vi "FtoC_SubVI.vi"(1 "Temperatura a Convertir":dbl) -> (0 "Temperatura Convertida":dbl)   [LabVIEW 2013]
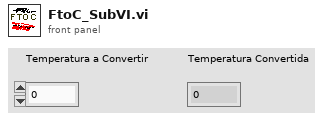
[diagram p1: front panel]
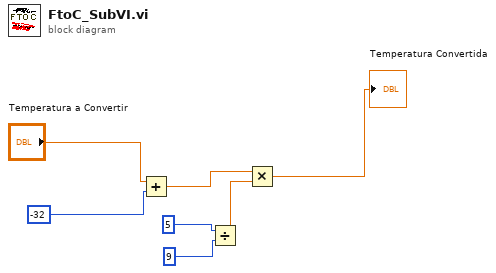
[diagram p0: block diagram]
diagram:
  n1 = Add(x="Temperatura a Convertir", y=-32) -> (x+y=w2:dbl)
  n2 = Divide(x=5, y=9) -> (x/y=w5:dbl)
  n3 = Multiply(x=w2, y=w5) -> (x*y=→"Temperatura Convertida":dbl)
